vi "PrimaryAttackerShot_Init.vi"(0 "object in":refnum<class "PrimaryAttackerShot.lvclass">, 5 "error in (no error)":errorcluster) -> (14 "object out":refnum<class "PrimaryAttackerShot.lvclass">, 19 "error out":errorcluster)   [LabVIEW 2023, in "PrimaryAttackerShot.lvclass"]
uses:
  PrimaryAttackerShot.lvclass
  C:/Users/ebert/Documents/codes/SSL/repo/SSL_AI/NewSTP/Evaluators/Evaluator_class/Evaluator.lvclass
  Criteria/OpenAngleToGoal_class/OpenAngleToGoal.lvclass
  C:/Users/ebert/Documents/codes/SSL/repo/SSL_AI/NewSTP/Criteria/Criterion_class/Criterion.lvclass
  Criteria/BallInterception_class/BallInterception.lvclass
  Criteria/OutOfGoalieArea_class/OutOfGoalieArea.lvclass
  Evaluator_class/Evaluator.lvclass
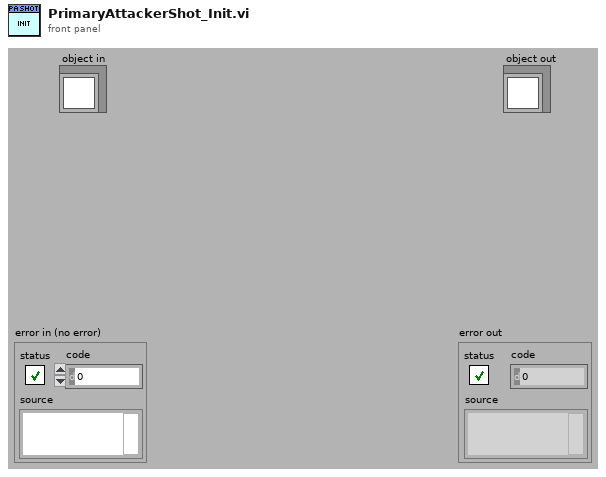
[diagram p1: front panel]
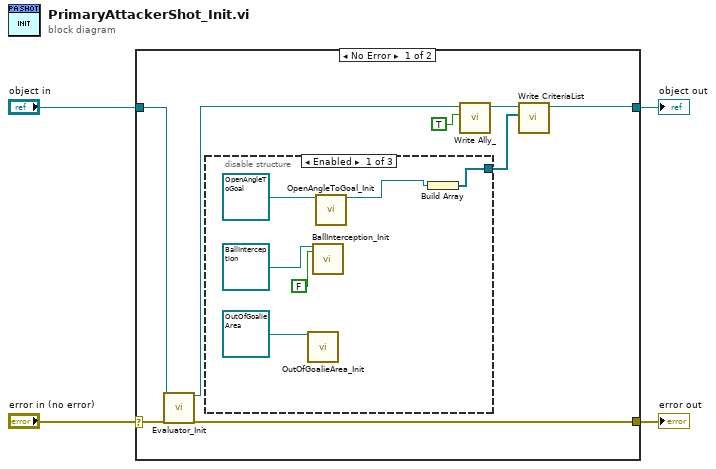
[diagram p0: block diagram]
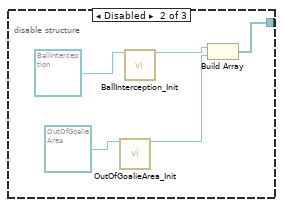
[diagram p2: hidden frame]
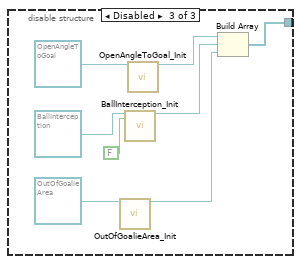
[diagram p3: hidden frame]
diagram:
  n1 = case shown="No Error" "error in (no error)" {
    selector: "error in (no error)" -> [w12 w32]
    tunnel: [w6 w33] -> w4
    tunnel: "object in" -> [w9 w33]
    tunnel: [w11 w32] -> w1
    frame No Error {
      n2 = call "Evaluator_Init.vi"("object in"=w9, "error in (no error)"=w12) -> ("object out"=w5:refnum<class "PrimaryAttackerShot.lvclass">, "error out"=w11:errorcluster)  [unwired: 16 in]
      n3 = disable-structure shown="Enabled" {
        disable-tunnel: [w13 w23 w30] -> w7
        frame Enabled {
          n4 = call "OutOfGoalieArea_Init.vi"("object in"=refnum<class "OutOfGoalieArea.lvclass"> refnum ("OutOfGoalieArea")) -> ()  [unwired: 17 in, 2 out]
          n5 = call "BallInterception_Init.vi"("object in"=refnum<class "BallInterception.lvclass"> refnum ("BallInterception"), "Pass?"=FALSE) -> ()  [unwired: 16 in, 2 out]
          n6 = call "OpenAngleToGoal_Init.vi"("object in"=refnum<class "OpenAngleToGoal.lvclass"> refnum ("OpenAngleToGoal")) -> ("object out"=w14:refnum<class "OpenAngleToGoal.lvclass">)  [unwired: 17 in, 1 out]
          n7 = Build Array(w14) -> (w13:refnum<class "OpenAngleToGoal.lvclass">[])
        }
        frame Disabled {
          n8 = call "OutOfGoalieArea_Init.vi"("object in"=refnum<class "OutOfGoalieArea.lvclass"> refnum ("OutOfGoalieArea")) -> ("object out"=w19:refnum<class "OutOfGoalieArea.lvclass">)  [unwired: 17 in, 1 out]
          n9 = call "BallInterception_Init.vi"("object in"=refnum<class "BallInterception.lvclass"> refnum ("BallInterception")) -> ("object out"=w22:refnum<class "BallInterception.lvclass">)  [unwired: 17 in, 1 out]
          n10 = Build Array(w22, w19) -> (w23:refnum<class "Criterion.lvclass">[])
        }
        frame Disabled {
          n11 = call "OutOfGoalieArea_Init.vi"("object in"=refnum<class "OutOfGoalieArea.lvclass"> refnum ("OutOfGoalieArea")) -> ("object out"=w25:refnum<class "OutOfGoalieArea.lvclass">)  [unwired: 17 in, 1 out]
          n12 = call "BallInterception_Init.vi"("object in"=refnum<class "BallInterception.lvclass"> refnum ("BallInterception"), "Pass?"=FALSE) -> ("object out"=w28:refnum<class "BallInterception.lvclass">)  [unwired: 16 in, 1 out]
          n13 = call "OpenAngleToGoal_Init.vi"("object in"=refnum<class "OpenAngleToGoal.lvclass"> refnum ("OpenAngleToGoal")) -> ("object out"=w24:refnum<class "OpenAngleToGoal.lvclass">)  [unwired: 17 in, 1 out]
          n14 = Build Array(w24, w28, w25) -> (w30:refnum<class "Criterion.lvclass">[])
        }
      }
      n15 = call-dynamic "Write Ally_.vi"("Ally?"=TRUE, "Evaluator in"=w5) -> ("Evaluator out"=w8:refnum<class "PrimaryAttackerShot.lvclass">)  [unwired: 8 in, 1 out]
      n16 = call-dynamic "Write CriteriaList.vi"("CriteriaList"=w7, "Evaluator in"=w8) -> ("Evaluator out"=w6:refnum<class "PrimaryAttackerShot.lvclass">)  [unwired: 8 in, 1 out]
    }
    frame Error {
    }
  }
  "object out" <- w4
  "error out" <- w1
